vi "Generate Vector Statements.vi"(0 "RFFE Command in":refnum<class "RFFE Command.lvclass">, 11 "error in (no error)":errorcluster) -> (4 "RFFE Command out":refnum<class "RFFE Command.lvclass">, 6 "Vector Statements":string[](array[string]), 15 "error out":errorcluster)   [LabVIEW 2018, in "MIPI RFFE API.lvlib" / "RFFE Command.lvclass"]
uses:
  RFFE Command.lvclass
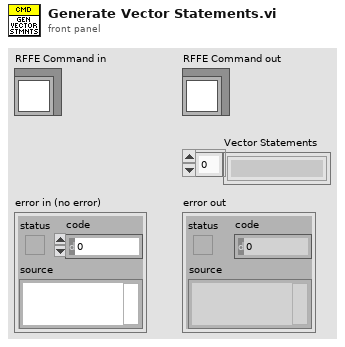
[diagram p1: front panel]
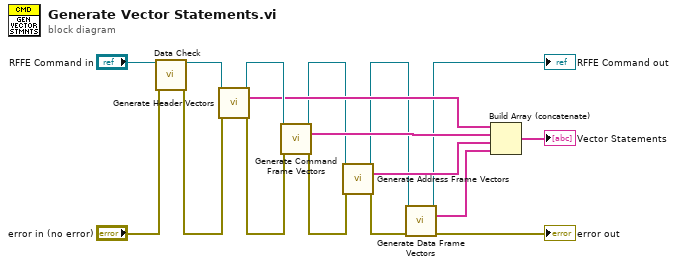
[diagram p0: block diagram]
diagram:
  n1 = call-dynamic "Data Check.vi"("RFFE Command in"="RFFE Command in", "error in (no error)"="error in (no error)") -> ("RFFE Command out"=w10:refnum<class "RFFE Command.lvclass">, "error out"=w9:errorcluster)  [unwired: 12 in]
  n2 = call-dynamic "Generate Header Vectors.vi"("RFFE Command in"=w10, "error in (no error)"=w9) -> ("RFFE Command out"=w14:refnum<class "RFFE Command.lvclass">, "Header Vectors"=w13:string[], "error out"=w12:errorcluster)  [unwired: 11 in]
  n3 = call-dynamic "Generate Command Frame Vectors.vi"("RFFE Command in"=w14, "error in (no error)"=w12) -> ("RFFE Command out"=w7:refnum<class "RFFE Command.lvclass">, "Command Frame Vectors"=w11:string[], "error out"=w6:errorcluster)  [unwired: 11 in]
  n4 = call-dynamic "Generate Address Frame Vectors.vi"("RFFE Command in"=w7, "error in (no error)"=w6) -> ("RFFE Command out"=w4:refnum<class "RFFE Command.lvclass">, "Address Frame Vectors"=w8:string[], "error out"=w5:errorcluster)  [unwired: 11 in]
  n5 = call-dynamic "Generate Data Frame Vectors.vi"("RFFE Command in"=w4, "error in (no error)"=w5) -> ("RFFE Command out"=→"RFFE Command out":refnum<class "RFFE Command.lvclass">, "Data Frame Vectors"=w2:string[], "error out"=→"error out":errorcluster)  [unwired: 11 in]
  n6 = Build Array (concatenate)(w13, w11, w8, w2) -> (→"Vector Statements":string[])
